vi "_Calculate Duration.vi"(1 "Method":i32[][](array[numeric])=[[0, 10, 3000, 100], [0, 4, 2000, 100], [0, 10, 1000, 100]]) -> (0 "RunTime(mS)":i32=50400)   [LabVIEW 2012]
panel:
  out "TotalExptRan":i32=24
  # "StartT (mS)"
  # "#of Cycle"
  # "CycleT (mS)"
  # "Expt 1"
  # "Expt 2"
  # "Expt 3"
  # "Expt 4"
  # "Expt 5"
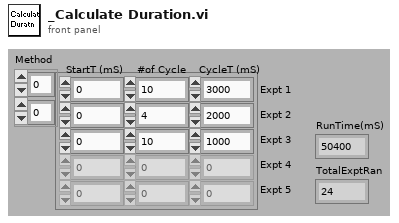
[diagram p1: front panel]
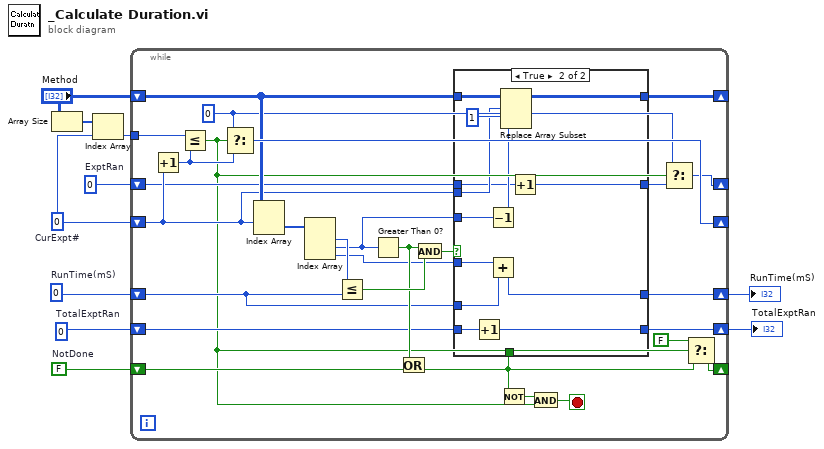
[diagram p0: block diagram]
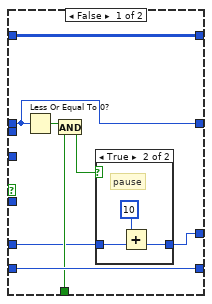
[diagram p2: hidden frame]
diagram:
  w1 = 0  # ExptRan
  w4 = 0  # TotalExptRan
  w7 = 0  # CurExpt#
  w9 = FALSE  # NotDone
  w10 = 0  # RunTime(mS)
  n1 = Array Size(array="Method") -> (size(s)=w6:i32[])
  n2 = Index Array(array=w6, index=w7) -> (element=w5:i32)
  n3 = while {
    shift-right: [w27] -> _
    shift-left: "Method" -> [w28]
    shift-right: [w15] -> w2
    shift-left: w10 -> [w23]
    shift-right: [w12] -> _
    shift-left: w9 -> [w36]
    shift-right: [w32] -> _
    shift-left: w7 -> [w24]
    tunnel: w5 -> [w34]
    shift-right: [w21] -> w3
    shift-left: w4 -> [w22]
    shift-right: [w16] -> _
    shift-left: w1 -> [w18]
    stop <- w30 stop-if-true
    w19 = 0 ("t")
    n4 = Increment(x=w24) -> (x+1=w33:i32)
    n5 = Less Or Equal?(x=w34, y=w33) -> (x <= y?=w14:bool)
    n6 = Select(t=w19, s=w14, f=w33) -> (s? t:f=w32:i32)
    n7 = Index Array(array=w28, index (row)=w24) -> (element=w26:i32[])  [unwired: 1 in]
    n8 = Index Array(array=w26) -> (element #1=w38:i32, element #2=w25:i32, element #3=w20:i32)  [unwired: 3 in]
    n9 = Less Or Equal?(x=w38, y=w23) -> (x <= y?=w37:bool)
    n10 = Greater Than 0?(x=w25) -> (x > 0?=w35:bool)
    n11 = Or(x=w35, y=w36) -> (x .or. y?=w13:bool)
    n12 = And(x=w35, y=w37) -> (x .and. y?=w29:bool)
    n13 = case shown="True" w29 {
      tunnel: w28 -> [w46 w62]
      tunnel: [w46 w58] -> w27
      tunnel: w25 -> [_ w63]
      tunnel: w24 -> [_ w60]
      tunnel: w23 -> [w40 w54]
      tunnel: w22 -> [w45 w57]
      tunnel: [w45 w56] -> w21
      tunnel: w20 -> [_ w55]
      tunnel: [w39 w53] -> w15
      tunnel: w13 -> [w43 _]
      tunnel: w18 -> [w42 w52]
      tunnel: [w42 w51] -> w17
      frame False {
        n14 = Less Or Equal To 0?(x=w42) -> (x <= 0?=w44:bool)
        n15 = And(x=w44, y=w43) -> (x .and. y?=w41:bool)
        n16 = case shown="True" w41 {
          tunnel: w40 -> [w47 w50]
          tunnel: [w47 w48] -> w39
          frame False {
          }
          frame True {
            # "pause"
            n17 = Add(x=10, y=w50) -> (x+y=w48:i32)
          }
        }
      }
      frame True {
        n18 = Increment(x=w57) -> (x+1=w56:i32)
        n19 = Decrement(x=w63) -> (x-1=w59:i32)
        n20 = Add(x=w55, y=w54) -> (x+y=w53:i32)
        n21 = Replace Array Subset(array=w62, new element=w59, index (row)=w60, index (col)=1 ("index")) -> (w58:i32[][])
        n22 = Increment(x=w52) -> (x+1=w51:i32)
      }
    }
    n23 = Not(x=w13) -> (.not. x?=w31:bool)
    n24 = And(x=w31, y=w14) -> (x .and. y?=w30:bool)
    n25 = Select(t=w19, s=w14, f=w17) -> (s? t:f=w16:i32)
    n26 = Select(t=FALSE, s=w14, f=w13) -> (s? t:f=w12:bool)
  }
  "TotalExptRan" <- w3
  "RunTime(mS)" <- w2
